vi "isInitialized.vi"(8 "error in (no error)":errorcluster, 11 "MsgUserEventStopMechanism In":refnum<class "MsgQueueTaskChannel.lvclass">) -> (0 "error out":errorcluster, 2 "isInitRequired":bool, 3 "MsgUserEventStopMechanism Out":refnum<class "MsgQueueTaskChannel.lvclass">)   [LabVIEW 2023, in "TLC_Daemon.lvlib" / "MsgQueueTaskChannel.lvclass"]
doc: "Returns True if the StopMechanism requires initialization.\nThis is useful for handling both of the following cases:\n- Internal Initialization: The StopMechanism is initialized by the TaskController, which handles the entire lifecycle.\n- External Initialization: The StopMechanism is already initialized externally. This is used when you need to share the mechanism with other components (such as message queues).\n\nNote: Use external initialization carefully; the TaskController sends stopRequests, which may impact external code."
uses:
  MsgUETaskChannel/MsgQueueTaskChannel.lvclass
  MsgUETaskChannel/MsgQueueTaskChannel.lvclass/MsgQueueTaskChannel.ctl
  Ctrls/msg.ctl
  TLC_Daemon.lvlib
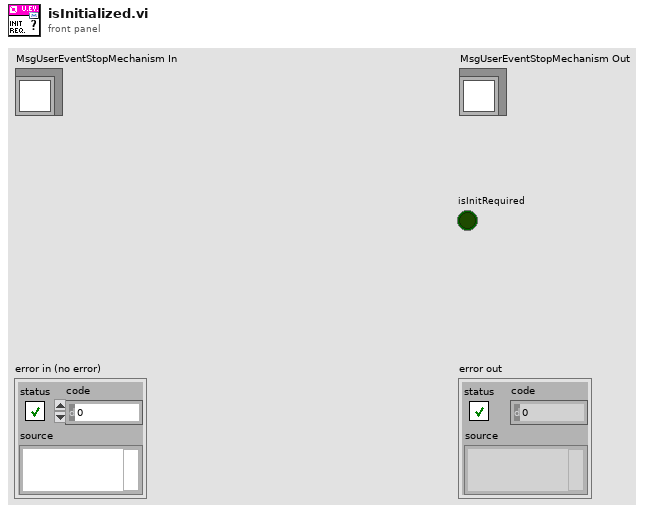
[diagram p1: front panel]
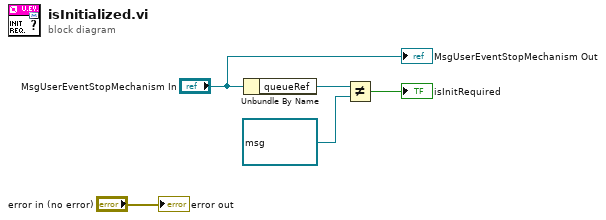
[diagram p0: block diagram]
diagram:
  n1 = Unbundle By Name("MsgUserEventStopMechanism In") -> ("queueRef"=w3:refnum<queue>)
  n2 = Not Equal?(x=w3, y=refnum<queue> refnum) -> (x != y?=→"isInitRequired":bool)
  "error out" <- "error in (no error)"
  "MsgUserEventStopMechanism Out" <- "MsgUserEventStopMechanism In"
